vi "viewerFrontEnd.vi"(8 "error in (no error)":errorcluster, 10 "defaultPath":path, 11 "ICSettingsViewer in":refnum<class "ICSettingsViewer.lvclass">) -> (0 "error out":errorcluster, 3 "ICSettingsViewer out":refnum<class "ICSettingsViewer.lvclass">)   [LabVIEW 2011, in "Views.lvlib" / "Camera.lvlib" / "ICSettingsViewer.lvclass"]
uses:
  ICSettingsViewer.lvclass
  Tools/SettingsEventManager/SettingsEventsManager.lvclass
  Tools/Filing/FileSystem/FileSystem.lvclass
  Tools/SettingsViewer/settingsViewer.lvclass
panel:
  out "start_trigger":string caption="Trigger Channel"
  in  "Upload":bool
  in  "image_number":i32 caption="Image Number"
  in  "Close":bool
  in  "Load":bool
  in  "Save":bool
  out "Triggering":bool
  in  "gain":i32(slide)=260 scale=260.0..1023.0
  in  "exposure":dbl(slide)=0.0064 min=0.0001 max=30.0 step=0.0001 scale=0.0..0.5
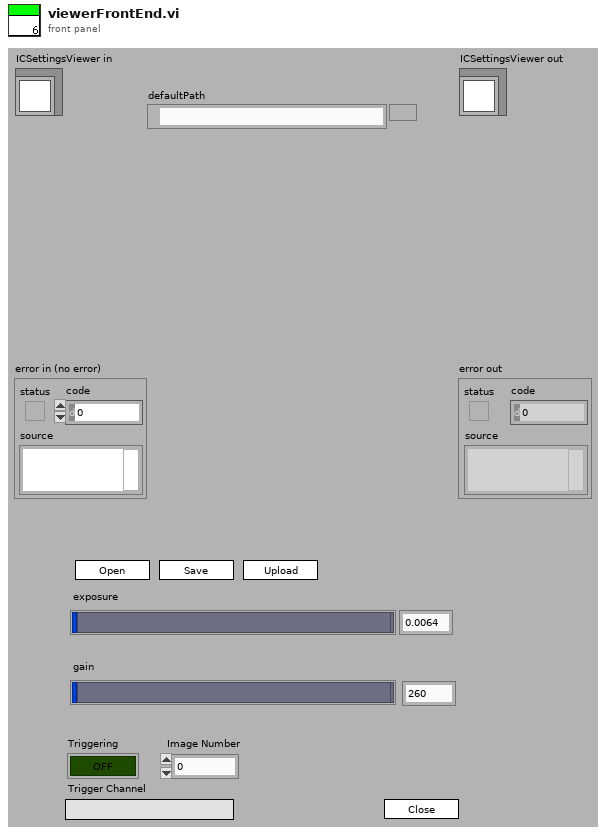
[diagram p1: front panel]
types:
  T1 = enum32{"Invalid", "Standard", "Closed", "Hidden", "Minimized", "Maximized"}
  T2 = enum16{"exposure time", "gain", "trigger mode", "image number"}
  T3 = cluster{"settingsFrontEndEvents":cluster{"loadSettingsFromPath":refnum<user-event>, "lookUpElementEvent":refnum<user-event>, "saveSettings":refnum<user-event>, "loadSettings":refnum<user-event>, "close":refnum<user-event>, "replaceElement":refnum<user-event>, "findParentNodes":refnum<user-event>, "createNode":refnum<user-event>}, "settingBackEndEvents":cluster{"defaultSettingsPathRequest":refnum<user-event>, "searchResultEvent":refnum<user-event>, "settingsSaved":refnum<user-event>, "settingsLoaded":refnum<user-event>, "foundParentNode":refnum<user-event>}}
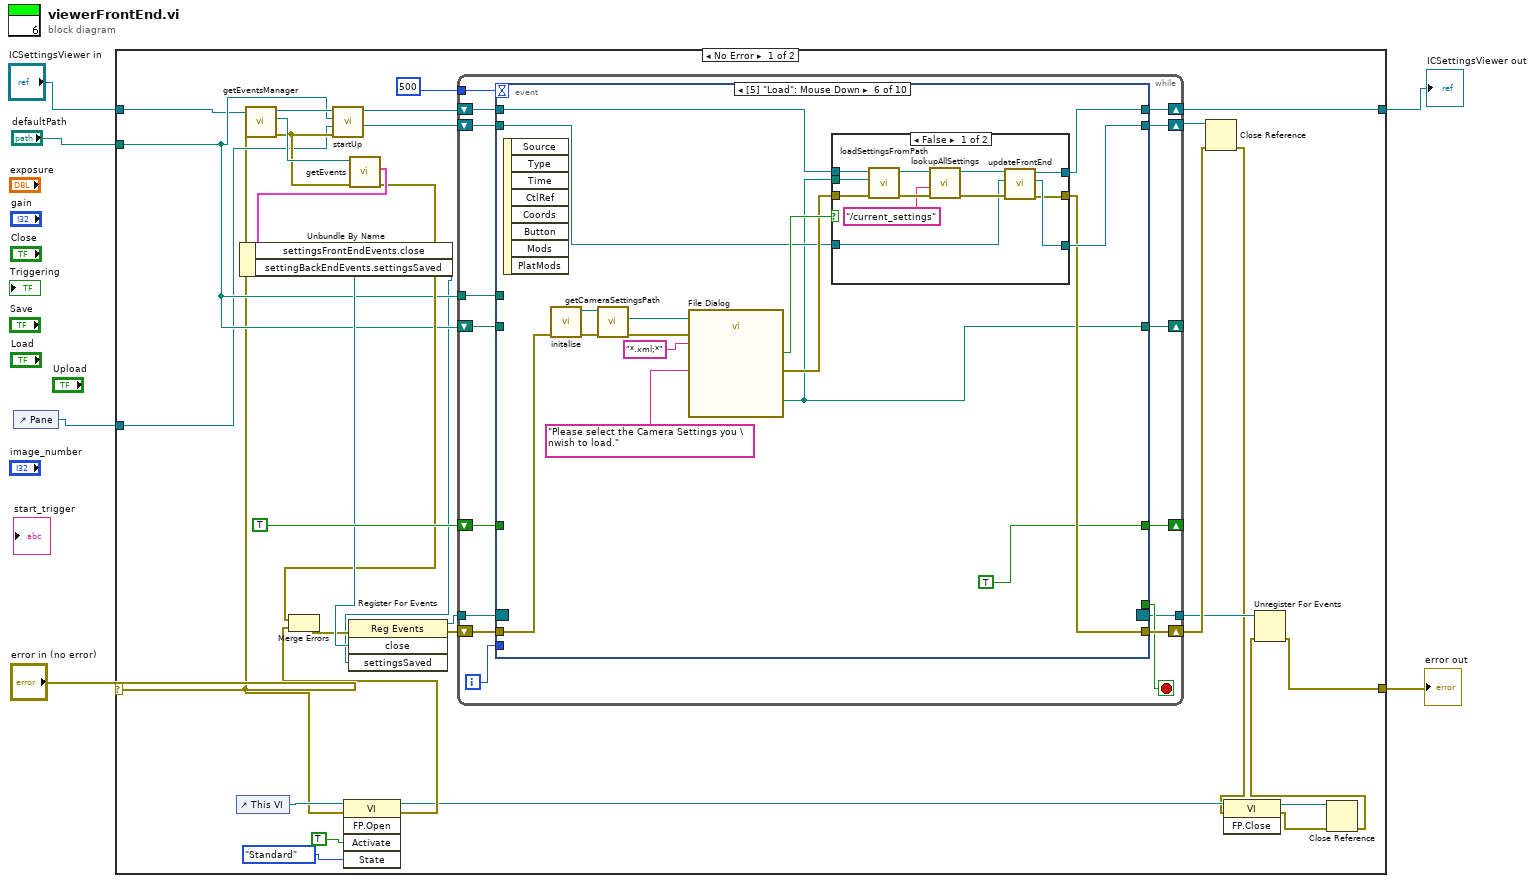
[diagram p0: block diagram]
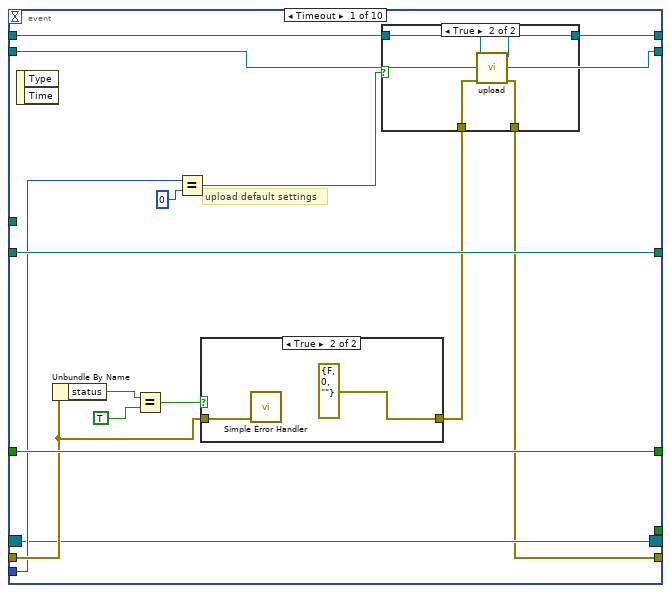
[diagram p2: hidden frame]
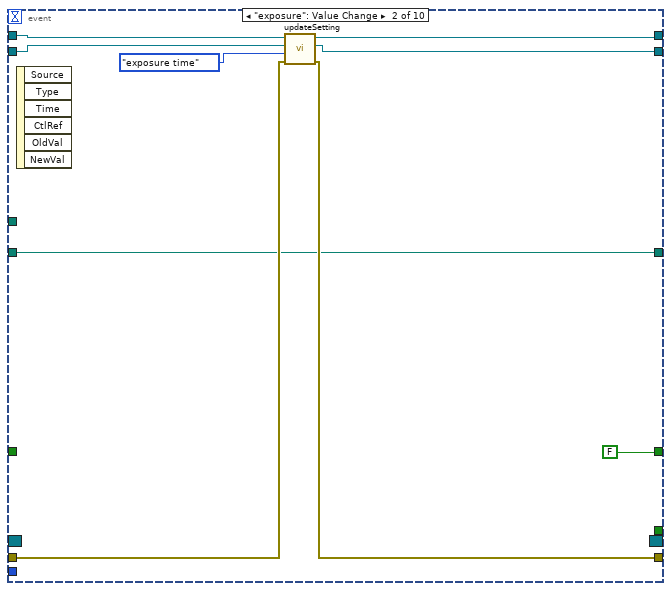
[diagram p5: hidden frame]
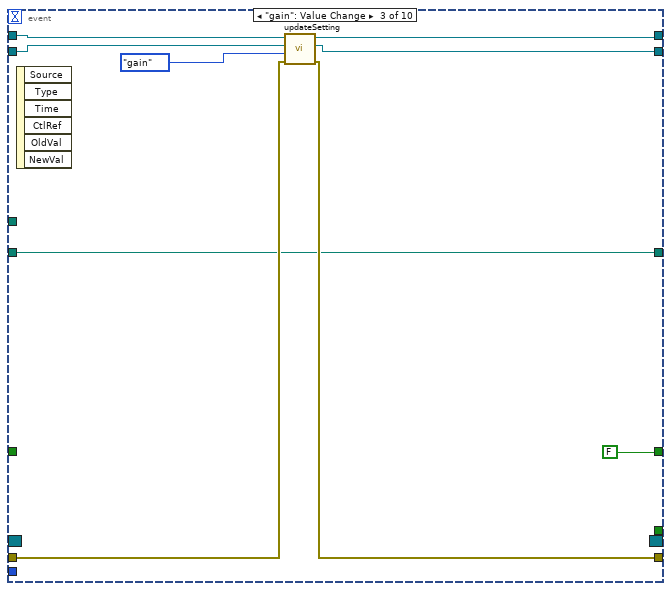
[diagram p6: hidden frame]
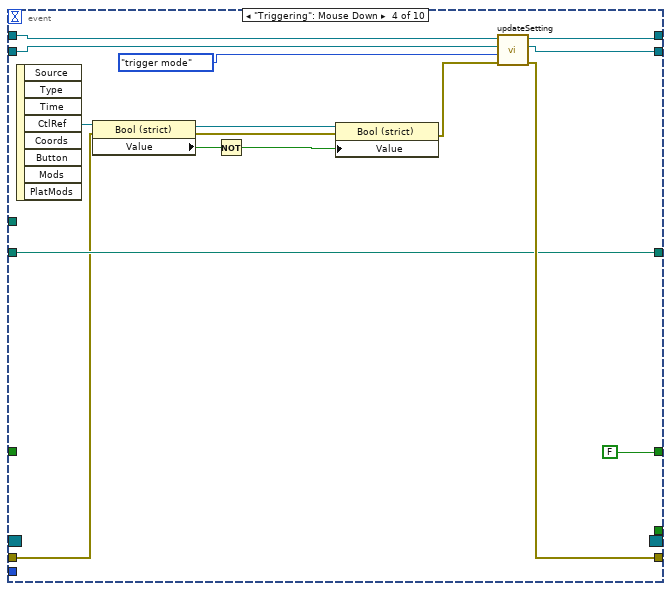
[diagram p7: hidden frame]
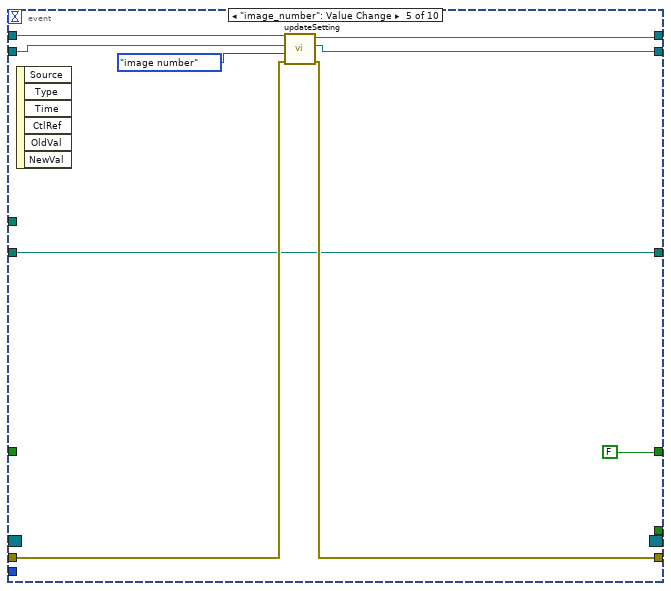
[diagram p8: hidden frame]
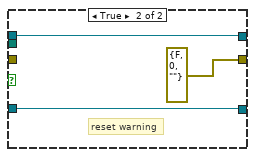
[diagram p9: hidden frame]
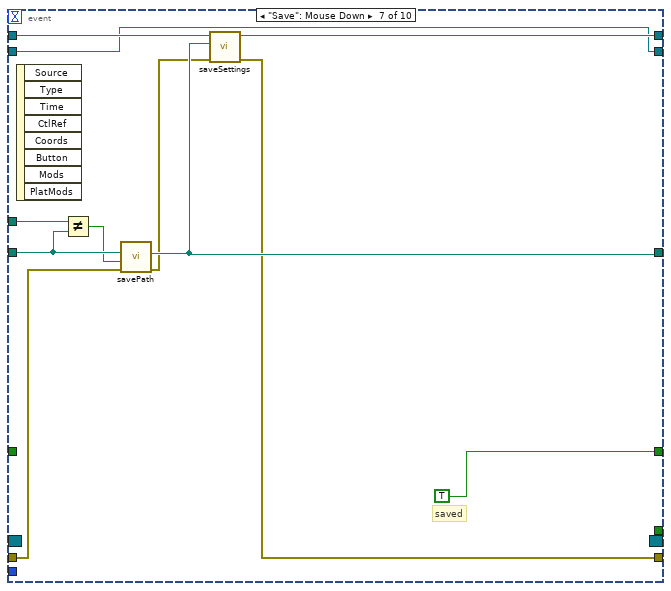
[diagram p10: hidden frame]
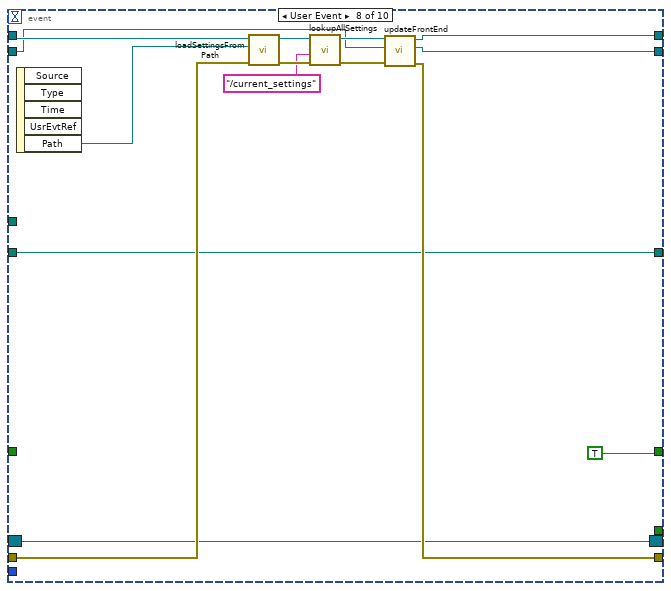
[diagram p11: hidden frame]
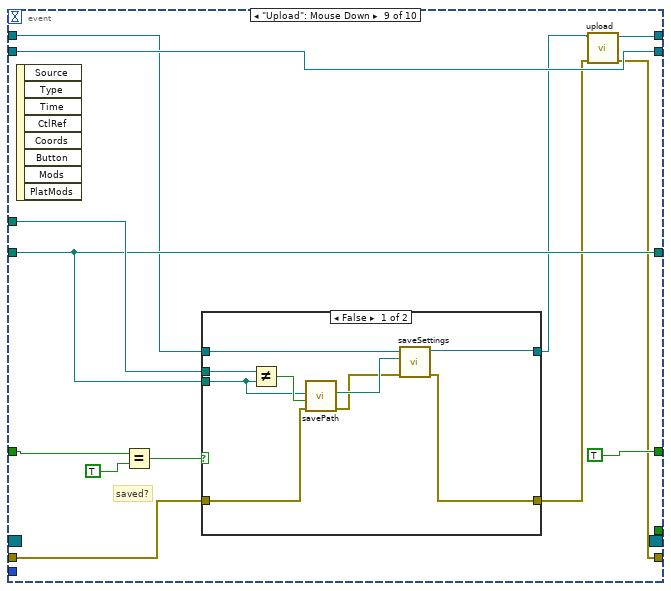
[diagram p12: hidden frame]
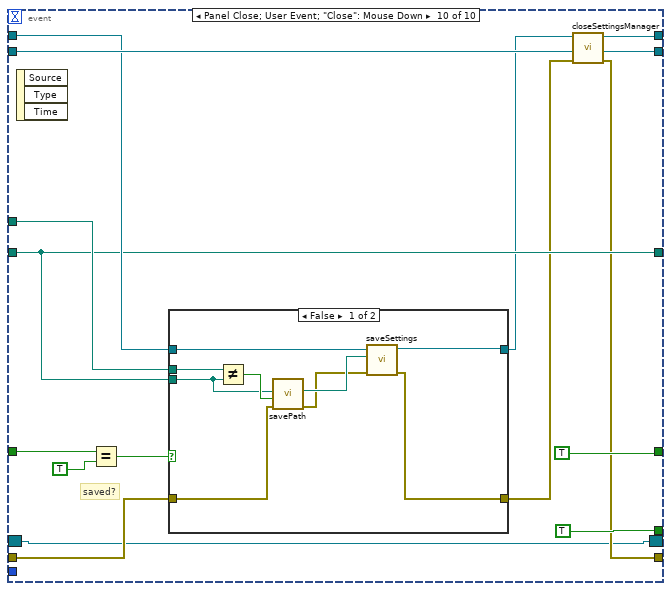
[diagram p14: hidden frame]
diagram:
  n1 = control-ref of="Pane"() -> (w2:refnum<vi>)
  n2 = case shown="No Error" "error in (no error)" {
    selector: "error in (no error)" -> [w11 w228]
    tunnel: "ICSettingsViewer in" -> [w8 w229]
    tunnel: "defaultPath" -> [w13 _]
    tunnel: [w38 w229] -> w4
    tunnel: [w27 w228] -> w3
    tunnel: w2 -> [w12 _]
    frame No Error {
      n3 = control-ref of="This VI"() -> (w26:refnum<vi>)
      n4 = call-dynamic "getEventsManager.vi"("error in (no error)"=w11, "SettingsViewer.lvclass in"=w8) -> ("error out"=w14:errorcluster, "Tools.lvlib:Settings.lvlib:SettingsEventsManager.lvclass"=w33:refnum<class "SettingsEventsManager.lvclass">, "SettingsViewer.lvclass out"=w15:refnum<class "ICSettingsViewer.lvclass">)  [unwired: 7 in]
      n5 = call "startUp.vi"("error in (no error)"=w14, "Pane"=w12, "Path"=w13, "ICSettingsViewer in"=w15) -> ("Pane out"=w9:refnum<vi>, "ICSettingsViewer out"=w10:refnum<class "ICSettingsViewer.lvclass">)  [unwired: 5 in, 1 out]
      n6 = invoke class="VI" method="FP.Open"(reference=w26, error in=w11, "Activate"=TRUE ("Activate?"), "State"=T1."Standard") -> (reference out=w20:refnum<vi>, error out=w21:errorcluster)  [unwired: 1 in, 3 out]
      n7 = call-dynamic "getEvents.vi"("error in (no error)"=w14, "SettingsEventsManager in"=w33) -> ("error out"=w22:errorcluster, "settingsEvents"=w32:T3)  [unwired: 7 in, 1 out]
      n8 = Unbundle By Name(w32) -> ("settingsFrontEndEvents.close"=w30:refnum<user-event>, "settingBackEndEvents.settingsSaved"=w7:refnum<user-event>)
      n9 = Merge Errors(w22, w21) -> (w23:errorcluster)
      n10 = register-events(error in=w23, w30, w7) -> (reference out=w29:refnum<event-registration>, error out=w31:errorcluster)  [unwired: 1 in]
      n11 = while {
        shift-right: [w53] -> w38
        shift-left: w10 -> [w54]
        shift-right: [w51] -> w35
        shift-left: w31 -> [w52]
        shift-right: [w49] -> w36
        shift-left: w9 -> [w50]
        shift-right: [w46] -> _
        shift-left: w13 -> [w47]
        tunnel: w13 -> [w45]
        shift-right: [w44] -> _
        shift-left: TRUE -> [w43]
        tunnel: 500 -> [w42]
        tunnel: w29 -> [w41]
        tunnel: [w40] -> w28
        i -> [w39]
        stop <- w48 stop-if-true
        n12 = event shown="[5] \"Load\": Mouse Down" {
          selector: w41 -> [w60 _ _ _ _ _ _ w165 _ w202]
          dyn-events: [w60 _ _ _ _ _ _ w165 _ w202] -> w40
          timeout: w42 -> [_ _ _ _ _ _ _ _ _ _]
          tunnel: [w58 w82 w91 w107 w115 w136 w154 w168 w180 w205] -> w53
          tunnel: w54 -> [w59 w87 w96 w111 w120 w127 w158 w172 w185 w211]
          tunnel: w52 -> [w63 w84 w93 w97 w117 w131 w162 w170 w183 w210]
          tunnel: [w56 w83 w92 w108 w116 w123 w155 w166 w178 w203] -> w51
          tunnel: w50 -> [w69 w86 w95 w110 w119 w125 w153 w169 w190 w216]
          tunnel: [w69 w81 w90 w106 w114 w124 w153 w167 w190 w216] -> w49
          tunnel: [_ _ _ _ _ _ _ _ _ TRUE] -> w48
          tunnel: w47 -> [w68 w80 w89 w105 w113 _ w160 w164 w186 w208]
          tunnel: [w68 w80 w89 w105 w113 w122 w157 w164 w186 w208] -> w46
          tunnel: w45 -> [_ _ _ _ _ _ w161 _ w187 w209]
          tunnel: [w67 FALSE FALSE FALSE FALSE TRUE TRUE TRUE TRUE TRUE] -> w44
          tunnel: w43 -> [w67 _ _ _ _ _ _ _ w182 w214]
          tunnel: w39 -> [w61 _ _ _ _ _ _ _ _ _]
          event Timeout {
            # "upload default settings"
            n13 = event-data() -> ()  [unwired: 1 in, 2 out]
            n14 = Unbundle By Name(w63) -> ("status"=w66:bool)
            n15 = Equal?(x=w66, y=TRUE) -> (x = y?=w64:bool)
            n16 = Equal?(x=w61, y=0) -> (x = y?=w55:bool)
            n17 = case shown="True" w64 {
              tunnel: [w76 errorcluster {"status"=FALSE, "code"=0, "source"=""} ("error out")] -> w57
              tunnel: w63 -> [w76 w77]
              frame False {
              }
              frame True {
                n18 = call <vilib>:"Simple Error Handler.vi"("error in (no error)"=w77) -> ()  [unwired: 4 in, 5 out]
              }
            }
            n19 = case shown="True" w55 {
              tunnel: w59 -> [w71 w75]
              tunnel: [w71 w74] -> w58
              tunnel: w57 -> [w70 w73]
              tunnel: [w70 w72] -> w56
              frame False {
              }
              frame True {
                n20 = call "upload.vi"("error in (no error)"=w73, "ICSettingsViewer in"=w75) -> ("error out"=w72:errorcluster, "ICSettingsViewer out"=w74:refnum<class "ICSettingsViewer.lvclass">)  [unwired: 8 in]
              }
            }
          }
          event "exposure": Value Change {
            n21 = event-data() -> ()  [unwired: 1 in, 6 out]
            n22 = call "updateSetting.vi"("error in (no error)"=w84, "Enum"=T2."exposure time", "Pane"=w86, "ICSettingsViewer in"=w87) -> ("error out"=w83:errorcluster, "Pane out"=w81:refnum<vi>, "ICSettingsViewer out"=w82:refnum<class "ICSettingsViewer.lvclass">)  [unwired: 5 in]
          }
          event "gain": Value Change {
            n23 = event-data() -> ()  [unwired: 1 in, 6 out]
            n24 = call "updateSetting.vi"("error in (no error)"=w93, "Enum"=T2."gain", "Pane"=w95, "ICSettingsViewer in"=w96) -> ("error out"=w92:errorcluster, "Pane out"=w90:refnum<vi>, "ICSettingsViewer out"=w91:refnum<class "ICSettingsViewer.lvclass">)  [unwired: 5 in]
          }
          event "Triggering": Mouse Down {
            n25 = event-data() -> ("CtlRef"=w103:refnum<vi>)  [unwired: 1 in, 7 out]
            n26 = property class="Bool (strict)"(reference=w103, error in=w97) -> (reference out=w101:refnum<vi>, error out=w100:errorcluster, "Value"=w102:bool)
            n27 = Not(x=w102) -> (.not. x?=w98:bool)
            n28 = property class="Bool (strict)"(reference=w101, error in=w100, "Value"=w98) -> (error out=w99:errorcluster)  [unwired: 1 out]
            n29 = call "updateSetting.vi"("error in (no error)"=w99, "Enum"=T2."trigger mode", "Pane"=w110, "ICSettingsViewer in"=w111) -> ("error out"=w108:errorcluster, "Pane out"=w106:refnum<vi>, "ICSettingsViewer out"=w107:refnum<class "ICSettingsViewer.lvclass">)  [unwired: 5 in]
          }
          event "image_number": Value Change {
            n30 = event-data() -> ()  [unwired: 1 in, 6 out]
            n31 = call "updateSetting.vi"("error in (no error)"=w117, "Enum"=T2."image number", "Pane"=w119, "ICSettingsViewer in"=w120) -> ("error out"=w116:errorcluster, "Pane out"=w114:refnum<vi>, "ICSettingsViewer out"=w115:refnum<class "ICSettingsViewer.lvclass">)  [unwired: 5 in]
          }
          event "Load": Mouse Down {
            n32 = event-data() -> ()  [unwired: 1 in, 8 out]
            n33 = call "initalise.vi"("error in (no error)"=w131) -> ("error out"=w132:errorcluster, "FileSystem out"=w133:refnum<class "FileSystem.lvclass">)  [unwired: 9 in]
            n34 = call-dynamic "getCameraSettingsPath.vi"("error in (no error)"=w132, "FileSystem.lvclass in"=w133) -> ("error out"=w129:errorcluster, "CameraSettingsPath"=w130:path)  [unwired: 7 in, 1 out]
            n35 = call "File Dialog"("start path"=w130, "prompt"="Please select the Camera Settings you \nwish to load.", "error in"=w129, "pattern (all files)"="*.xml;*") -> ("selected path"=w122:path, "cancelled"=w128:bool, "error out"=w126:errorcluster)  [unwired: 8 in, 1 out]
            n36 = case shown="False" w128 {
              tunnel: [w143 w151] -> w136
              tunnel: w127 -> [w142 w151]
              tunnel: w125 -> [w141 w150]
              tunnel: [w140 w150] -> w124
              tunnel: w126 -> [w139 _]
              tunnel: w122 -> [w138 _]
              tunnel: [w137 errorcluster {"status"=FALSE, "code"=0, "source"=""} ("error out")] -> w123
              frame False {
                n37 = call "loadSettingsFromPath.vi"("error in (no error)"=w139, "Path"=w138, "ICSettingsViewer in"=w142) -> ("error out"=w147:errorcluster, "ICSettingsViewer out"=w148:refnum<class "ICSettingsViewer.lvclass">)  [unwired: 7 in]
                n38 = call "lookupAllSettings.vi"("error in (no error)"=w147, "whichSettings"="/current_settings", "ICSettingsViewer in"=w148) -> ("error out"=w144:errorcluster, "ICSettingsViewer out"=w145:refnum<class "ICSettingsViewer.lvclass">)  [unwired: 7 in]
                n39 = call "updateFrontEnd.vi"("error in (no error)"=w144, "Pane"=w141, "ICSettingsViewer in"=w145) -> ("error out"=w137:errorcluster, "Pane out"=w140:refnum<vi>, "ICSettingsViewer out"=w143:refnum<class "ICSettingsViewer.lvclass">)  [unwired: 6 in]
              }
              frame True {
                # "reset warning"
              }
            }
          }
          event "Save": Mouse Down {
            # "saved"
            n40 = event-data() -> ()  [unwired: 1 in, 8 out]
            n41 = Not Equal?(x=w161, y=w160) -> (x != y?=w159:bool)
            n42 = call "savePath.vi"("error in (no error)"=w162, "overwrite?"=w159, "Path  in"=w160) -> ("error out"=w156:errorcluster, "Path out"=w157:path)  [unwired: 6 in, 1 out]
            n43 = call "saveSettings.vi"("error in (no error)"=w156, "Path"=w157, "ICSettingsViewer in"=w158) -> ("error out"=w155:errorcluster, "ICSettingsViewer out"=w154:refnum<class "ICSettingsViewer.lvclass">)  [unwired: 7 in]
          }
          event User Event {
            n44 = event-data() -> ("Path"=w171:path)  [unwired: 1 in, 4 out]
            n45 = call "loadSettingsFromPath.vi"("error in (no error)"=w170, "Path"=w171, "ICSettingsViewer in"=w172) -> ("error out"=w176:errorcluster, "ICSettingsViewer out"=w177:refnum<class "ICSettingsViewer.lvclass">)  [unwired: 7 in]
            n46 = call "lookupAllSettings.vi"("error in (no error)"=w176, "whichSettings"="/current_settings", "ICSettingsViewer in"=w177) -> ("error out"=w173:errorcluster, "ICSettingsViewer out"=w174:refnum<class "ICSettingsViewer.lvclass">)  [unwired: 7 in]
            n47 = call "updateFrontEnd.vi"("error in (no error)"=w173, "Pane"=w169, "ICSettingsViewer in"=w174) -> ("error out"=w166:errorcluster, "Pane out"=w167:refnum<vi>, "ICSettingsViewer out"=w168:refnum<class "ICSettingsViewer.lvclass">)  [unwired: 6 in]
          }
          event "Upload": Mouse Down {
            # "saved?"
            n48 = event-data() -> ()  [unwired: 1 in, 8 out]
            n49 = Equal?(x=w182, y=TRUE) -> (x = y?=w188:bool)
            n50 = case shown="False" w188 {
              tunnel: w185 -> [w195 w201]
              tunnel: [w196 w201] -> w181
              tunnel: w183 -> [w192 w200]
              tunnel: [w191 w200] -> w179
              tunnel: w187 -> [w194 _]
              tunnel: w186 -> [w193 _]
              frame False {
                n51 = Not Equal?(x=w194, y=w193) -> (x != y?=w199:bool)
                n52 = call "savePath.vi"("error in (no error)"=w192, "overwrite?"=w199, "Path  in"=w193) -> ("error out"=w197:errorcluster, "Path out"=w198:path)  [unwired: 6 in, 1 out]
                n53 = call "saveSettings.vi"("error in (no error)"=w197, "Path"=w198, "ICSettingsViewer in"=w195) -> ("error out"=w191:errorcluster, "ICSettingsViewer out"=w196:refnum<class "ICSettingsViewer.lvclass">)  [unwired: 7 in]
              }
              frame True {
              }
            }
            n54 = call "upload.vi"("error in (no error)"=w179, "ICSettingsViewer in"=w181) -> ("error out"=w178:errorcluster, "ICSettingsViewer out"=w180:refnum<class "ICSettingsViewer.lvclass">)  [unwired: 8 in]
          }
          event Panel Close; User Event; "Close": Mouse Down {
            # "saved?"
            n55 = event-data() -> ()  [unwired: 1 in, 3 out]
            n56 = Equal?(x=w214, y=TRUE) -> (x = y?=w212:bool)
            n57 = case shown="False" w212 {
              tunnel: w211 -> [w221 w227]
              tunnel: [w222 w227] -> w206
              tunnel: w210 -> [w218 w226]
              tunnel: [w217 w226] -> w204
              tunnel: w209 -> [w220 _]
              tunnel: w208 -> [w219 _]
              frame False {
                n58 = Not Equal?(x=w220, y=w219) -> (x != y?=w225:bool)
                n59 = call "savePath.vi"("error in (no error)"=w218, "overwrite?"=w225, "Path  in"=w219) -> ("error out"=w223:errorcluster, "Path out"=w224:path)  [unwired: 6 in, 1 out]
                n60 = call "saveSettings.vi"("error in (no error)"=w223, "Path"=w224, "ICSettingsViewer in"=w221) -> ("error out"=w217:errorcluster, "ICSettingsViewer out"=w222:refnum<class "ICSettingsViewer.lvclass">)  [unwired: 7 in]
              }
              frame True {
              }
            }
            n61 = call "closeSettingsManager.vi"("error in (no error)"=w204, "ICSettingsViewer in"=w206) -> ("error out"=w203:errorcluster, "ICSettingsViewer out"=w205:refnum<class "ICSettingsViewer.lvclass">)  [unwired: 8 in]
          }
        }
      }
      n62 = Close Reference(reference=w36, error in (no error)=w35) -> (error out=w19:errorcluster)
      n63 = invoke class="VI" method="FP.Close"(reference=w20, error in=w19) -> (reference out=w18:refnum<vi>, error out=w17:errorcluster)  [unwired: 1 in, 1 out]
      n64 = Close Reference(reference=w18, error in (no error)=w17) -> (error out=w16:errorcluster)
      n65 = Unregister For Events(event registration refnum=w28, error in=w16) -> (error out=w27:errorcluster)
    }
    frame Error {
    }
  }
  "error out" <- w3
  "ICSettingsViewer out" <- w4
